vi "Clear DTC.vi"(6 "Action":T3, 8 "error in":errorcluster, 9 "Address (ALL)":string="ALL", 10 "Address Lookup Table":variant, 11 "connection info":T1) -> (0 "error out":errorcluster, 2 "Address Lookup Table Out":variant, 3 "connection info":T1)   [LabVIEW 2023, in "J1939 Host Automation API.lvlib"]
uses:
  J1939 Host Automation API.lvlib
  <vilib>/NI/STM/TCP/TCP Connection Info.ctl
  <vilib>/NI/STM/SubVIs/MetaDataElement.ctl
  Addon/Addon Shared/Types/DTC_Action.ctl
  Addon/Addon Shared/J1939 Addon Shared.lvlib
  <vilib>/NI/STM/NI STM.lvlib
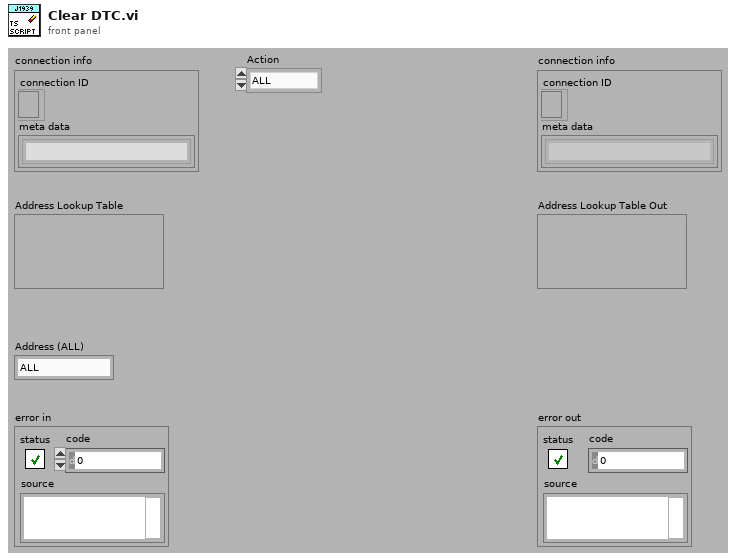
[diagram p1: front panel]
types:
  T1 = typedef "NI STM.lvlib/TCP Connection Info.ctl" = cluster{"connection ID":refnum<k5>, "meta data":T2[]}
  T2 = typedef "NI STM.lvlib/MetaDataElement.ctl" = string
  T3 = typedef "J1939 Addon Shared.lvlib/DTC_Action.ctl" = enum16{"ALL", "ACTIVE", "INACTIVE"}
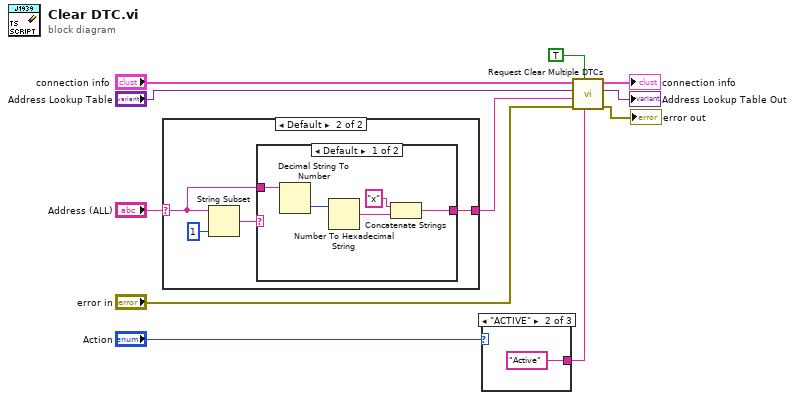
[diagram p0: block diagram]
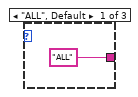
[diagram p4: hidden frame]
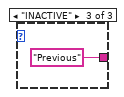
[diagram p5: hidden frame]
diagram:
  n1 = case shown="Default" "Address (ALL)" {
    selector: "Address (ALL)" -> [w12 w14]
    tunnel: [w12 w13] -> w1
    frame "ALL" {
    }
    frame Default {
      n2 = String Subset(string=w14, length (rest)=1 ("length (rest)")) -> (substring=w15:string)  [unwired: 1 in]
      n3 = case shown="Default" w15 {
        tunnel: w14 -> [w21 w22]
        tunnel: [w17 w22] -> w13
        frame Default {
          n4 = Decimal String To Number(string=w21) -> (number=w20:i32)  [unwired: 2 in, 1 out]
          n5 = Number To Hexadecimal String(2:w20) -> (0:w19:string)  [unwired: 1 in]
          n6 = Concatenate Strings("x" ("string"), w19) -> (w17:string)
        }
        frame "x" {
        }
      }
    }
  }
  n7 = case shown="\"ACTIVE\"" "Action" {
    tunnel: ["ALL" ("TLA (ALL)") "Active" ("TLA (ALL)") "Previous" ("TLA (ALL)")] -> w7
    frame "ALL", Default {
    }
    frame "ACTIVE" {
    }
    frame "INACTIVE" {
    }
  }
  n8 = call "Request Clear Multiple DTCs.vi"("Command"=w7, "Ignore Response"=TRUE, "error in"="error in", "Address"=w1, "Lookup Table"="Address Lookup Table", "connection info"="connection info") -> ("error out"=→"error out":errorcluster, "Lookup Table"=→"Address Lookup Table Out":variant, "connection info"=→"connection info":T1)  [unwired: 2 in, 1 out]
